vi "SimpleFuncGen.vi"(8 "reset signal":bool, 9 "#s":dbl, 10 "Fs":dbl, 11 "Outputs":T1) -> (3 "Array":waveform(dbl)[](array[waveform]))   [LabVIEW 2023]
uses:
  <vilib>/measure/NI_MABase.lvlib
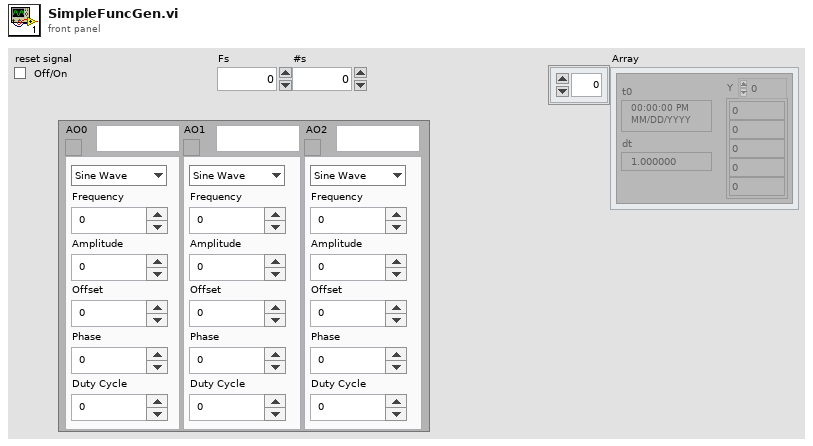
[diagram p1: front panel]
types:
  T1 = cluster{"AO0":cluster{"signal type":enum16{"Sine Wave", "Triangle Wave", "Square Wave", "Sawtooth Wave"}, "Frequency":dbl, "Amplitude":dbl, "Offset":dbl, "Phase":dbl, "Duty Cycle":dbl}, "AO0Enable":bool, "AO1":cluster{"signal type":enum16{"Sine Wave", "Triangle Wave", "Square Wave", "Sawtooth Wave"}, "Frequency":dbl, "Amplitude":dbl, "Offset":dbl, "Phase":dbl, "Duty Cycle":dbl}, "AO1Enable":bool, "AO2":cluster{"signal type":enum16{"Sine Wave", "Triangle Wave", "Square Wave", "Sawtooth Wave"}, "Frequency":dbl, "Amplitude":dbl, "Offset":dbl, "Phase":dbl, "Duty Cycle":dbl}, "AO3Enable":bool, "AO0Name":string, "AO1Name":string, "AO2Name":string}
  T2 = cluster{"signal type":enum16{"Sine Wave", "Triangle Wave", "Square Wave", "Sawtooth Wave"}, "Frequency":dbl, "Amplitude":dbl, "Offset":dbl, "Phase":dbl, "Duty Cycle":dbl}
  T3 = cluster{"signal type":enum16{"Sine Wave", "Triangle Wave", "Square Wave", "Sawtooth Wave"}, "Frequency":dbl, "Amplitude":dbl, "Offset":dbl, "Phase":dbl, "Duty Cycle":dbl}[]
  T4 = enum16{"Sine Wave", "Triangle Wave", "Square Wave", "Sawtooth Wave"}
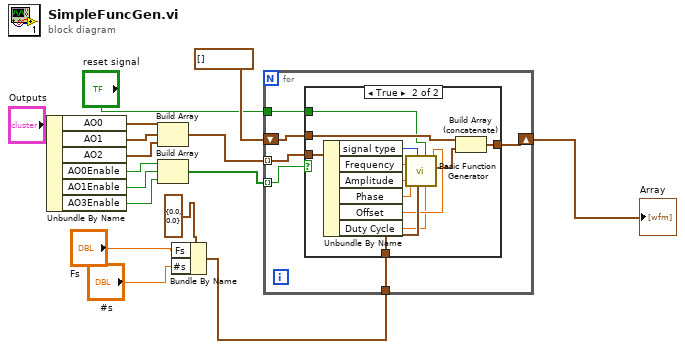
[diagram p0: block diagram]
diagram:
  n1 = Unbundle By Name("Outputs") -> ("AO0"=w12:T2, "AO1"=w11:T2, "AO2"=w10:T2, "AO0Enable"=w6:bool, "AO1Enable"=w5:bool, "AO3Enable"=w4:bool)
  n2 = Build Array(w12, w11, w10) -> (w9:T3)
  n3 = Build Array(w6, w5, w4) -> (w3:bool[])
  n4 = Bundle By Name(cluster=cluster{"Fs":dbl, "#s":dbl} {"Fs"=0.0, "#s"=0.0} ("sampling info"), "Fs"="Fs", "#s"="#s") -> (w14:cluster{"Fs":dbl, "#s":dbl})
  n5 = for {
    tunnel: w14 -> [w22]
    tunnel: w9 -> [w21] mode=indexing
    tunnel: w3 -> [w20] mode=indexing
    shift-right: [w19] -> w16
    shift-left: waveform(dbl)[] [] -> [w18]
    tunnel: "reset signal" -> [w17]
    n6 = case shown="True" w20 {
      tunnel: w22 -> [_ w35]
      tunnel: w21 -> [_ w34]
      tunnel: [w23 w26] -> w19
      tunnel: w18 -> [w23 w25]
      tunnel: w17 -> [_ w24]
      frame False {
      }
      frame True {
        n7 = Unbundle By Name(w34) -> ("signal type"=w33:T4, "Frequency"=w32:dbl, "Amplitude"=w31:dbl, "Phase"=w30:dbl, "Offset"=w29:dbl, "Duty Cycle"=w28:dbl)
        n8 = call <vilib>:"Basic Function Generator.vi"("offset"=w29, "square wave duty cycle (%)"=w28, "reset signal"=w24, "sampling info"=w35, "signal type"=w33, "phase"=w30, "amplitude"=w31, "frequency"=w32) -> ("signal out"=w27:waveform(dbl))  [unwired: 1 in, 2 out]
        n9 = Build Array (concatenate)(w25, w27) -> (w26:waveform(dbl)[])
      }
    }
  }
  "Array" <- w16
